vi "Side - Signal Generator.vi"() -> ()   [LabVIEW 2018]
uses:
  <vilib>/Platform/TimedLoop/XDataNode/timing_clust.ctl
  <vilib>/Platform/TimedLoop/XDataNode/nitl_modes.ctl
  <vilib>/Platform/TimedLoop/XDataNode/wakeup.ctl
  <vilib>/express/express analysis/Spectral/Block/exnSpectralBlock spectral measurements power poly.vi
  <vilib>/express/express analysis/Spectral/Block/exnSpectralBlock spectral measurements power DDT.vi
  <vilib>/express/express analysis/Spectral/XNode/ExpressSpectralMeasurementsBlockNode.xnode
  <vilib>/platform/TimedLoop/XDataNode/XDataNode.xnode
  <vilib>/myRIO/Express VI/Onboard IO/AO/AO Express VI.xnode
  <vilib>/Platform/TimedLoop/XDataNode/XDNodeRunTimeDep.lvlib
panel:
  in  "Offset":dbl
  in  "Frequency":dbl=10.1
  in  "Phase":dbl
  out "Sine":dynamicdata(graph)
  in  "Amplitude":dbl=1.0
  out "FTT Graph":dynamicdata(graph)
  in  "Sampling Rate (Hz)":dbl=1000.0 format="%0.2f"
  in  "# of Samples":i32=100
  in  "Simulate Noise":bool
  in  "Noise Type":u16(ring) items=["Uniform White Noise", "Gaussian White Noise", "Periodic Random Noise", "Gamma Noise", "Poisson Noise", "Binomial Noise", "Bernoulli Noise", "MLS Sequence "]
  in  "Signal Type":u16(ring) items=["Sine", "Square", "Triangle", "Sawtooth", "DC"]
  in  "Generate Data in Real Time":bool=TRUE
  in  "Play the Sound":bool
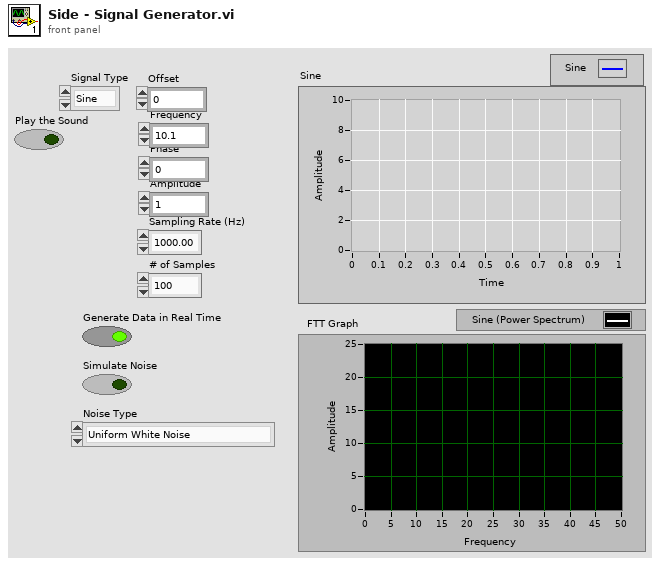
[diagram p1: front panel]
types:
  T1 = typedef "XDNodeRunTimeDep.lvlib/timing_clust.ctl" = cluster{"Expected End [f-1]":u64, "Actual End [f-1]":u64, "Finished Late? [f-1]":bool, "Expected End [i-1]":u64, "Actual End [i-1]":u64, "Finished Late? [i-1]":bool, "Expected Start [i]":u64, "Actual Start [i]":u64, "Expected Start [f]":u64, "Actual Start [f]":u64, "Source Name":string, "Structure Name":string, "Period":i64, "Deadline":i64, "Offset":i64, "Start":i64, "Priority":i32, "Timeout":i32, "Mode":T2, "Wakeup Reason":T3, "Error":errorcluster, "Source Type":string, "Secondary Source Type":string, "Global End Time":u64, "Global Start Time":u64, "Frame Duration":u64, "Iteration Duration":u64, "Assigned CPU":i32, "I/O Scan Engine Mode":u32}
  T2 = typedef "XDNodeRunTimeDep.lvlib/nitl_modes.ctl" = enum32{"No Change", "Process missed periods, maintain original phase", "Discard missed periods, maintain original phase", "Process missed periods, ignore original phase", "Discard missed periods, ignore original phase"}
  T3 = typedef "XDNodeRunTimeDep.lvlib/wakeup.ctl" = enum32{"Normal", "Aborted", "Asynchronous wakeup", "Timing source error", "Timed loop error", "Timeout"}
  T4 = cluster{"averaging mode":u16, "weighting mode":u16, "number of averages":u32}
  T5 = cluster{"dB On (F)":bool, "unwrap phase (F)":bool, "convert to degree (F)":bool}
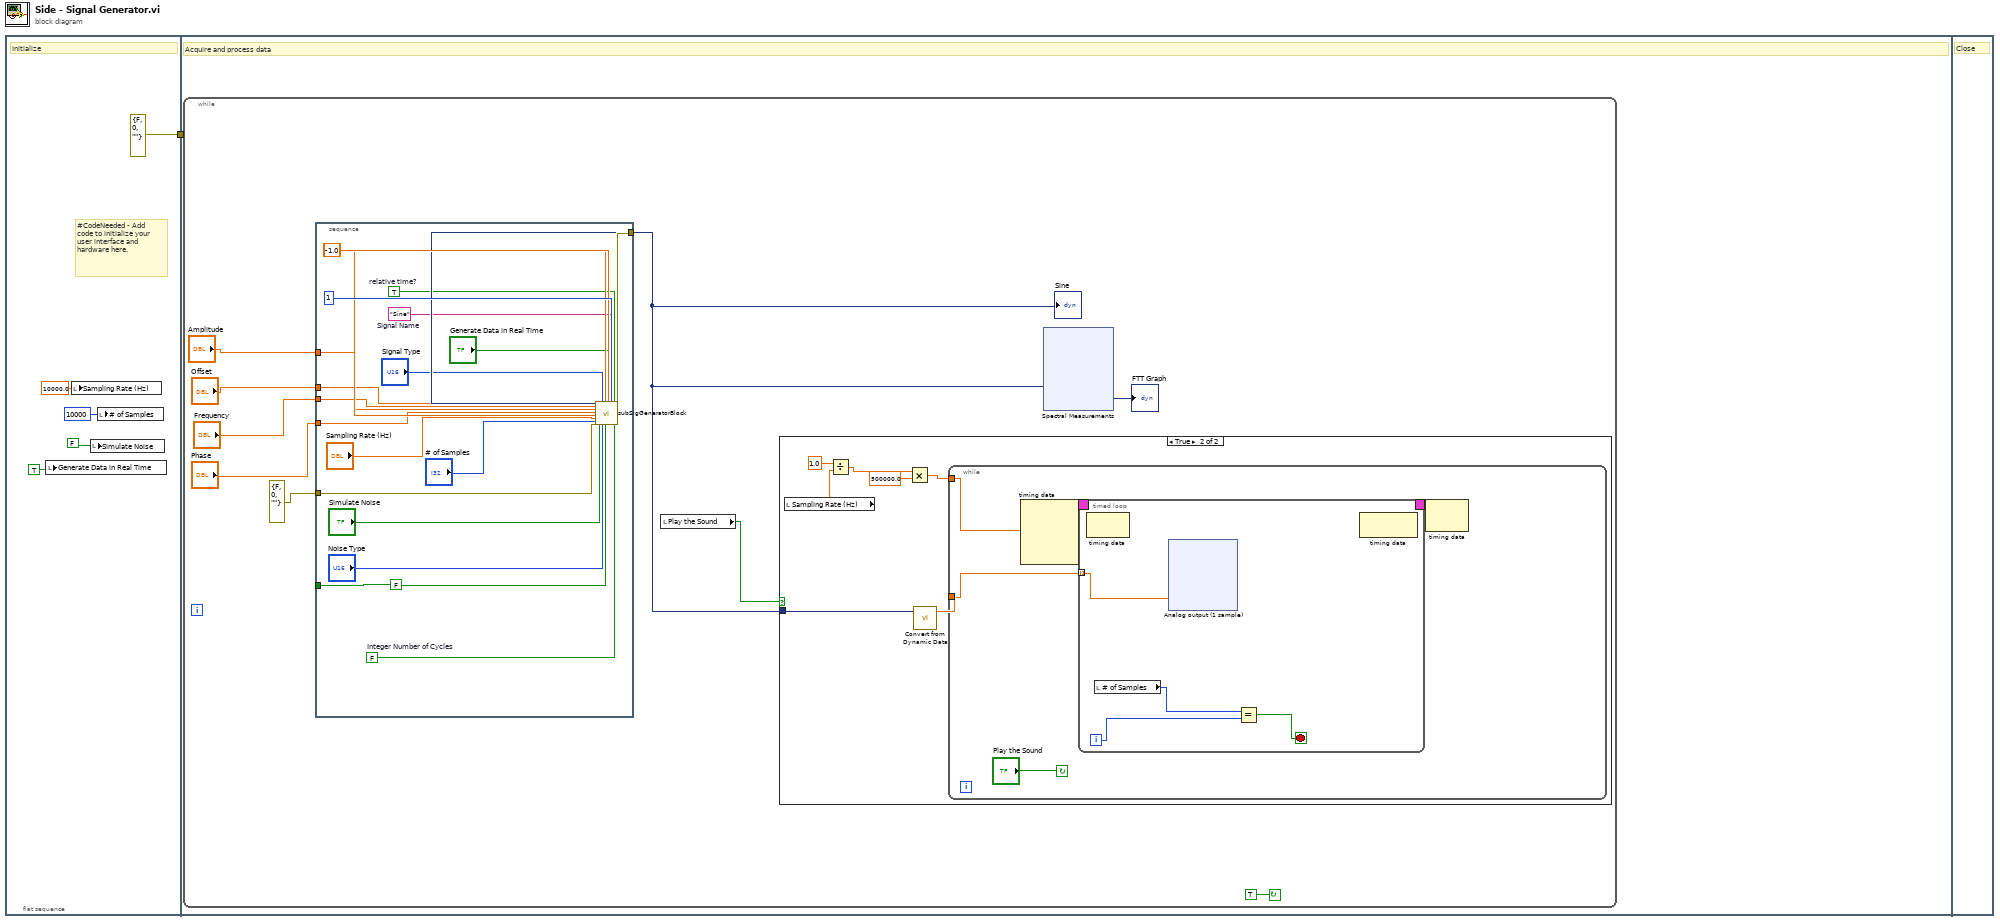
[diagram p0: block diagram]
diagram:
  n1 = flat-sequence {
    tunnel: [errorcluster {"status"=FALSE, "code"=0, "source"=""} ("error in (no error)")] -> w1
    tunnel: w1 -> [_]
    frame #0 {
      # "#CodeNeeded - Add code to initialize your user interface and hardware here."
      # "Initialize"
      n2 = local write "Generate Data in Real Time"(TRUE ("Generate Data in Real Time")) -> ()
      n3 = local write "Sampling Rate (Hz)"(10000.0 ("Sampling Rate (Hz)")) -> ()
      n4 = local write "Simulate Noise"(FALSE ("Noise")) -> ()
      n5 = local write "# of Samples"(10000 ("# of Samples")) -> ()
    }
    frame #1 {
      # "Acquire and process data"
      n6 = while {
        stop <- TRUE continue-if-true
        n7 = stacked-sequence {
          tunnel: "Offset" -> [w39]
          tunnel: FALSE ("Reset Signal") -> [w48]
          tunnel: [w52] -> w8
          tunnel: "Frequency" -> [w40]
          tunnel: "Amplitude" -> [w41]
          tunnel: "Phase" -> [w42]
          tunnel: errorcluster {"status"=FALSE, "code"=0, "source"=""} ("error in (no error)") -> [w46]
          tunnel: [w53] -> _
          frame #0 {
            w59 = FALSE  # Integer Number of Cycles
            w51 = TRUE  # relative time?
            w50 = "Sine"  # Signal Name
            n8 = call <vilib>:"subSigGeneratorBlock.vi"("Offset"=w39, "Frequency"=w40, "Amplitude"=w41, "Phase"=w42, "Duty Cycle (%)"=50.0, "Sampling Rate (Hz)"="Sampling Rate (Hz)", "# of Samples"="# of Samples", "error in (no error)"=w46, "Noise"="Simulate Noise", "Generate"="Signal Type", "Noise Ring"="Noise Type", "Reset Signal"=w48, "Noise Amplitude"=0.6 ("Noise amplitude"), "Generate Data in Real Time"="Generate Data in Real Time", "Seed Number"=-1.0, "Signal Name"=w50, "trials"=1 ("Trials"), "relative time?"=w51, "Integer Number of Cycles"=w59) -> ("Signal"=w52:dynamicdata, "error out"=w53:errorcluster)  [unwired: 7 in]
          }
        }
        "Sine" <- w8
        n9 = local read "Play the Sound"() -> (w7:bool)
        n10 = case shown="True" w7 {
          tunnel: w8 -> [_ w23]
          frame False {
          }
          frame True {
            n11 = local read "Sampling Rate (Hz)"() -> (w20:dbl)
            n12 = Divide(x=1.0, y=w20) -> (x/y=w19:dbl)
            n13 = Multiply(x=w19, y=500000.0) -> (x*y=w17:dbl)
            n14 = call "Convert from Dynamic Data"("Dynamic Data Type"=w23) -> ("Array"=w22:dbl[])  [unwired: 3 in]
            n15 = while {
              tunnel: w22 -> [w26]
              tunnel: w17 -> [w24]
              stop <- "Play the Sound" continue-if-true
              n16 = node-c288(w24) -> (w28:T1)  [unwired: 3 in]
              n17 = timed-loop {
                timing: w28 -> [_]
                timing-out: [_] -> w27
                tunnel: w26 -> [w29] mode=indexing
                i -> [w30]
                stop <- w31 stop-if-true
                n18 = node-c288() -> ()  [unwired: 1 in, 1 out]
                n19 = local read "# of Samples"() -> (w32:i32)
                n20 = xnode "Analog output (1 sample)"("V+ Input\nV+ Input (AudioOut/Left)"=w29) -> ()  [unwired: 1 in, 1 out]
                n21 = Equal?(x=w32, y=w30) -> (x = y?=w31:bool)
                n22 = node-c288() -> ()  [unwired: 1 in, 1 out]
              }
              n23 = node-c288(w27) -> ()  [unwired: 1 out]
            }
          }
        }
        n24 = xnode "Spectral Measurements"("Signals"=w8) -> ("Power Spectrum"=→"FTT Graph":dynamicdata)  [unwired: 1 in, 1 out]
      }
    }
    frame #2 {
      # "Close"
    }
  }
